vi "Init FPGA.vi"(8 "error in (no error)":errorcluster, 11 "FPGA Ref":T1) -> (0 "error out":errorcluster, 3 "FPGA Ref OUT":T1)   [LabVIEW 2013]
uses:
  <vilib>/rvi/interface/nirviReadWriteControl/nirviReadWriteControl.xnode
  Controls/FPGA_Reference.ctl
  FPGA/bitfiles/TI sbRIO PWM (FPGA) v1.0.lvbitx
  <vilib>/rvi/errors/niLvFpgaMergeErrorWithErrorCode.vi
  <vilib>/rvi/errors/niLvFpgaAdjustHostInterfaceError.vi
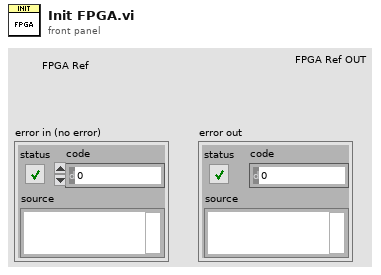
[diagram p1: front panel]
types:
  T1 = typedef "FPGA_Reference.ctl" = refnum<k20>
  T2 = cluster{"Divide Value":u8, "Transfer Length (bits)":u8, "CS Asserted Polarity":bool, "Clock Polarity (CPOL)":bool, "Clock Phase (CPHA)":bool, "Lengthen MISO Setup":bool, "Direction Change Bit":u8, "MOSI Starts as Output":bool, "Tristatable MOSI":bool}
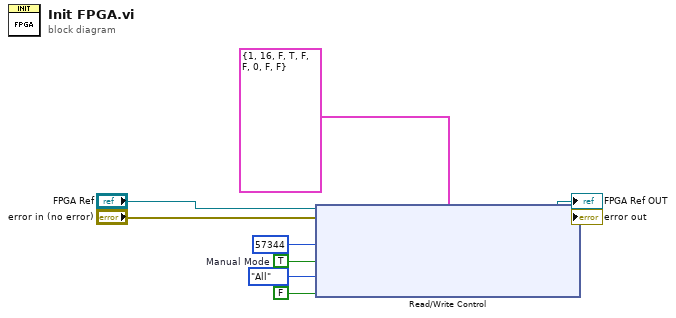
[diagram p0: block diagram]
diagram:
  w4 = TRUE  # Manual Mode
  n1 = xnode "Read/Write Control"("FPGA VI Reference In"="FPGA Ref", "error in"="error in (no error)", "ADC SPI Settings"=T2 {"Divide Value"=1, "Transfer Length (bits)"=16, "CS Asserted Polarity"=FALSE, "Clock Polarity (CPOL)"=TRUE, "Clock Phase (CPHA)"=FALSE, "Lengthen MISO Setup"=FALSE, "Direction Change Bit"=0, "MOSI Starts as Output"=FALSE, "Tristatable MOSI"=FALSE} ("Master Settings"), "ADC Data In"=u64 57344 ("data to write"), "ADC Manual"=w4, "ADC CS Mode"=enum16{"All", "CS0", "CS1"}."All" ("Mode"), "ADC Trigger"=FALSE ("nx-100 Trigger")) -> ("FPGA VI Reference Out"=→"FPGA Ref OUT":T1, "error out"=→"error out":errorcluster)
